vi "Pre Launch Init.vi"(11 "Launch in":refnum<class "Launch.lvclass">) -> (0 "error out":errorcluster, 3 "Launch out":refnum<class "Launch.lvclass">)   [LabVIEW 2020, in "PreLaunch Error.lvlib" / "Launch.lvclass"]
doc: "Override this VI to do any initialization that you need to have happen during Launch. This VI is guaranteed to finish before Launch Actor.vi returns to its caller, whereas any initialization that you do in Actor Core.vi may not have finished running when the caller starts sending messages. This VI is invoked from within the actor, not the caller, which means that any refnums created in this VI will have the same lifetime as \"Actor Core.vi\". The actor object will already be populated with both its queue and its caller's queue, so the two protected accessor methods \"Get Queue For Sending To Caller.vi\" and \"Get Queue For Sending To Self.vi\" may be used if necessary."
uses:
  Launch.lvclass
  Core/ActorFramework/Actor/Actor.lvclass
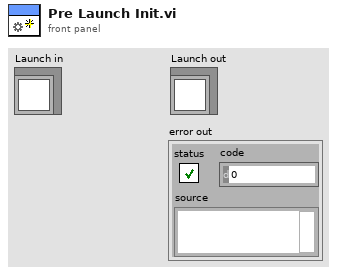
[diagram p1: front panel]
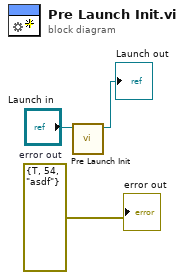
[diagram p0: block diagram]
diagram:
  w1 = errorcluster {"status"=TRUE, "code"=54, "source"="asdf"}  # error out
  n1 = call-parent "Pre Launch Init.vi"("Actor in"="Launch in") -> ("Actor out"=→"Launch out":refnum<class "Launch.lvclass">)  [unwired: 9 in, 1 out]
  "error out" <- w1
